vi "MultiExpB.vi"() -> ()   [LabVIEW 2017]
uses:
  001597bf-7838-4f65-85b7-67713ed17df7.vi
  Experiment/ExpGet.vi
  Expose/Labview/Core/ExposeInvokeMethod.vi
  <userlib>/_OpenG.lib/lvdata/lvdata.llb/Get Default Data from Variant__ogtk.vi
panel:
  in  "milliseconds to wait":u32=1000
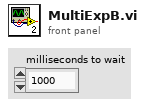
[diagram p1: front panel]
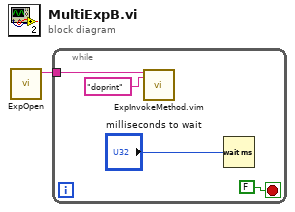
[diagram p0: block diagram]
diagram:
  n1 = call "ExpOpen.vi"() -> ("ExpID"=w1:string)  [unwired: 9 in, 2 out]
  n2 = while {
    tunnel: w1 -> [w4]
    stop <- FALSE stop-if-true
    n3 = call "ExpInvokeMethod.vim"("ExpID"=w4, "Method Name"="doprint") -> ()  [unwired: 15 in, 3 out]
    n4 = Wait (ms)(milliseconds to wait="milliseconds to wait") -> ()  [unwired: 1 out]
  }
